vi "AlliGator Get Destination Folder.vi"(8 "Error In":errorcluster, 9 "Current Data Set (-1: single)":i32=-1, 10 "Time-Series Paths":path[](array[path]), 11 "Single Data Point Path":path) -> (0 "Error Out":errorcluster, 1 "Data Point Name":string, 3 "Destination Folder path":path)   [LabVIEW 2021, in "AlliGator Files.lvlib"]
doc: "Returns the folder in which the current dataset is saved."
uses:
  AlliGator Files.lvlib
  Files/Files.lvlib
panel:
  # "see the AlliGator License on the block diagram (Ctrl+E or Window:Show Block Diagram)"
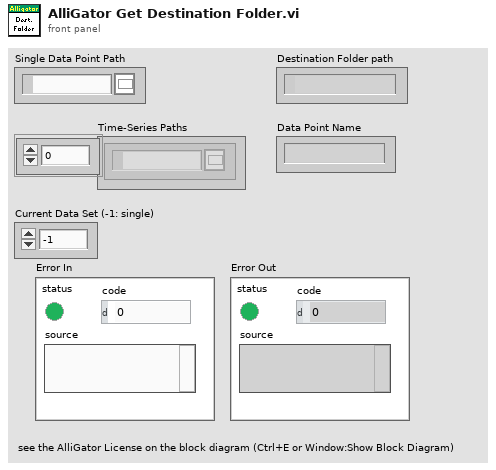
[diagram p1: front panel]
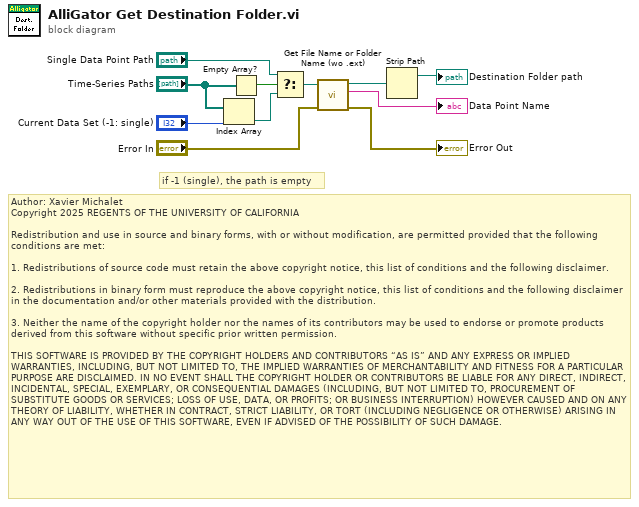
[diagram p0: block diagram]
diagram:
  # "Author: Xavier Michalet\nCopyright 2025 REGENTS OF THE UNIVERSITY OF CALIFORNIA\n\nRedistribution and use in source and binary forms, with or without modification, are permitted provided that the following conditions are met:\n\n1. Redistributions of source code must retain the above copyright notice, this list of conditions and the following disclaimer.\n\n2. Redistributions in binary form must reproduce the above copyright notice, this list of conditions and the following disclaimer in the documentation and/or other materials provided with the distribution.\n\n3. Neither the name of the copyright holder nor the names of its contributors may be used to endorse or promote products derived from this software without specific prior written permission.\n\nTHIS SOFTWARE IS PROVIDED BY THE COPYRIGHT HOLDERS AND CONTRIBUTORS “AS IS” AND ANY EXPRESS OR IMPLIED WARRANTIES, INCLUDING, BUT NOT LIMITED TO, THE IMPLIED WARRANTIES OF MERCHANTABILITY AND FITNESS FOR A PARTICULAR PURPOSE ARE DISCLAIMED. IN NO EVENT SHALL THE COPYRIGHT HOLDER OR CONTRIBUTORS BE LIABLE FOR ANY DIRECT, INDIRECT, INCIDENTAL, SPECIAL, EXEMPLARY, OR CONSEQUENTIAL DAMAGES (INCLUDING, BUT NOT LIMITED TO, PROCUREMENT OF SUBSTITUTE GOODS OR SERVICES; LOSS OF USE, DATA, OR PROFITS; OR BUSINESS INTERRUPTION) HOWEVER CAUSED AND ON ANY THEORY OF LIABILITY, WHETHER IN CONTRACT, STRICT LIABILITY, OR TORT (INCLUDING NEGLIGENCE OR OTHERWISE) ARISING IN ANY WAY OUT OF THE USE OF THIS SOFTWARE, EVEN IF ADVISED OF THE POSSIBILITY OF SUCH DAMAGE."
  # "if -1 (single), the path is empty"
  n1 = Index Array(array="Time-Series Paths", index="Current Data Set (-1: single)") -> (element=w8:path)
  n2 = Empty Array?(array="Time-Series Paths") -> (empty?=w6:bool)
  n3 = Select(t="Single Data Point Path", s=w6, f=w8) -> (s? t:f=w5:path)
  n4 = call "Get File Name or Folder Name (wo .ext).vi"("error in (no error)"="Error In", "input path"=w5) -> ("error out"=→"Error Out":errorcluster, "filename without extension"=→"Data Point Name":string, "dup path"=w4:path)  [unwired: 7 in]
  n5 = Strip Path(path=w4) -> (stripped path=→"Destination Folder path":path)  [unwired: 1 out]
